vi "DIAG_STM Get Meta Data (TCP).vi"(8 "error in":errorcluster, 11 "Connection Info":T1) -> (0 "error out":errorcluster, 2 "Meta data":T2[](array[typedef]), 3 "Connection Info Out":T1)   [LabVIEW 2015, in "Diagnostics Addon Engine.lvlib"]
doc: "Returns the meta data associated with the STM session."
uses:
  Diagnostics Addon Engine.lvlib
  stm_TCP Connection Info.ctl
  _SubVIs/stm_MetaDataElement.ctl
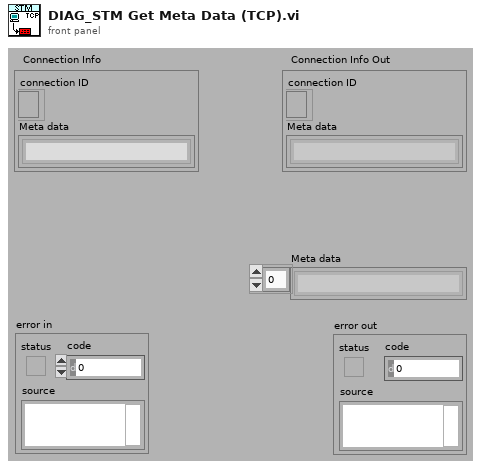
[diagram p1: front panel]
types:
  T1 = typedef "Diagnostics Addon Engine.lvlib/stm_TCP Connection Info.ctl" = cluster{"connection ID":refnum<k5>, "Meta data":T2[]}
  T2 = typedef "Diagnostics Addon Engine.lvlib/stm_MetaDataElement.ctl" = string
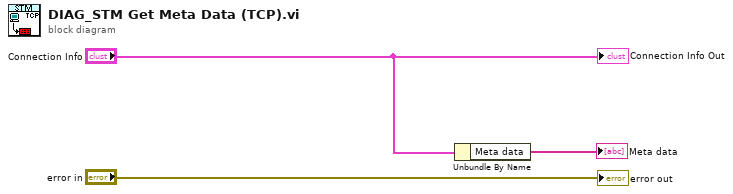
[diagram p0: block diagram]
diagram:
  n1 = Unbundle By Name("Connection Info") -> ("Meta data"=→"Meta data":T2[])
  "Connection Info Out" <- "Connection Info"
  "error out" <- "error in"
